vi "CU_estimateQuality.vi"(0 "Quality Measure in":T1, 5 "Confusion Matrix in":i32[][](array[numeric])) -> (7 "Classification Quality out":dbl)   [LabVIEW 2016, in "Classifier.lvlib"]
uses:
  Classifier.lvlib
  CU_ClassifierQualityMeasure.ctl
panel:
  # "This VI is a part of BCI Design library, http://www.ru-bci.org \nCopyright © 2020, Sotnikov Peter, All rights reserved. License: GNU GPLv3"
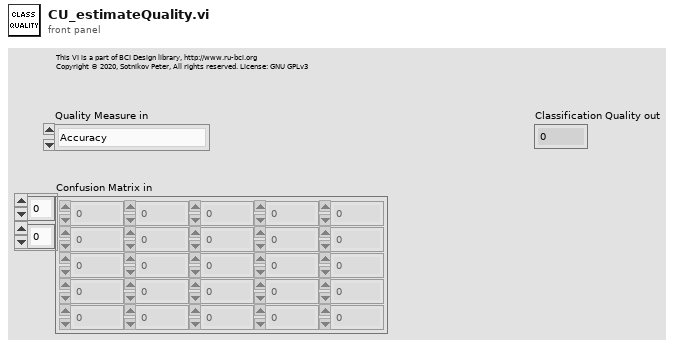
[diagram p1: front panel]
types:
  T1 = typedef "Classifier.lvlib/CU_ClassifierQualityMeasure.ctl" = enum16{"Accuracy", "Cohen's kappa"}
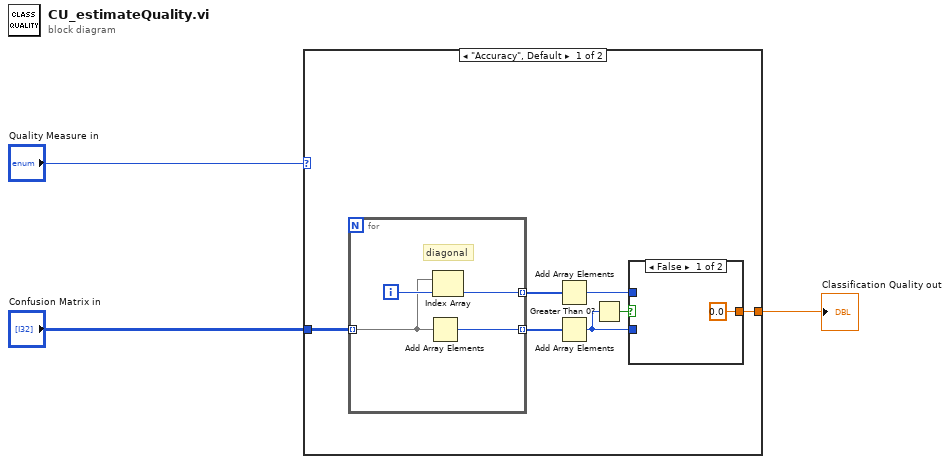
[diagram p0: block diagram]
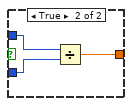
[diagram p2: hidden frame]
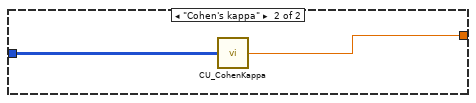
[diagram p3: hidden frame]
diagram:
  n1 = case shown="\"Accuracy\", Default" "Quality Measure in" {
    tunnel: "Confusion Matrix in" -> [w10 w20]
    tunnel: [w6 w19] -> w1
    frame "Accuracy", Default {
      n2 = for {
        tunnel: w10 -> [w17] mode=indexing
        tunnel: [w16] -> w9 mode=indexing
        tunnel: [w15] -> w8 mode=indexing
        i -> [w18]
        # "diagonal"
        n3 = Add Array Elements(numeric array=w17) -> (sum=w16:i32)
        n4 = Index Array(array=w17, index=w18) -> (element=w15:i32)
      }
      n5 = Add Array Elements(numeric array=w8) -> (sum=w7:i32)
      n6 = Add Array Elements(numeric array=w9) -> (sum=w5:i32)
      n7 = Greater Than 0?(x=w5) -> (x > 0?=w4:bool)
      n8 = case shown="False" w4 {
        tunnel: w5 -> [_ w12]
        tunnel: w7 -> [_ w13]
        tunnel: [0.0 w14] -> w6
        frame False {
        }
        frame True {
          n9 = Divide(x=w13, y=w12) -> (x/y=w14:dbl)
        }
      }
    }
    frame "Cohen's kappa" {
      n10 = call "CU_CohenKappa.vi"("Confusion Matrix"=w20) -> ("CohenKappa"=w19:dbl)  [unwired: 4 in]
    }
  }
  "Classification Quality out" <- w1
